vi "CheckValid.vi"(8 "error in (no error)":errorcluster, 11 "Cluster":T2) -> (0 "error out":errorcluster, 3 "Cluster 2":T1)   [LabVIEW 2019, in "lv-providershell-example2.lvlib"]
uses:
  lv-providershell-example2.lvlib
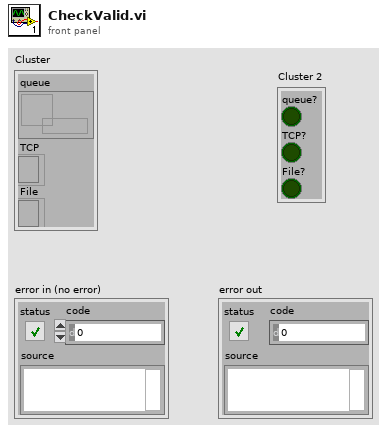
[diagram p1: front panel]
types:
  T1 = cluster{"queue?":bool, "TCP?":bool, "File?":bool}
  T2 = cluster{"queue":refnum<queue>, "TCP":refnum<k5>, "File":refnum<file>}
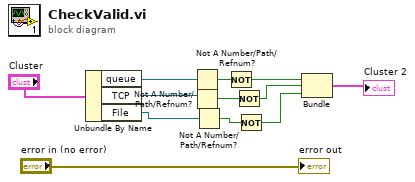
[diagram p0: block diagram]
diagram:
  n1 = Unbundle By Name("Cluster") -> ("queue"=w9:refnum<queue>, "TCP"=w8:refnum<k5>, "File"=w7:refnum<file>)
  n2 = Not A Number/Path/Refnum?(number/path/refnum=w9) -> (NaN/Path/Refnum?=w10:bool)
  n3 = Not A Number/Path/Refnum?(number/path/refnum=w8) -> (NaN/Path/Refnum?=w6:bool)
  n4 = Not A Number/Path/Refnum?(number/path/refnum=w7) -> (NaN/Path/Refnum?=w5:bool)
  n5 = Not(x=w10) -> (.not. x?=w4:bool)
  n6 = Not(x=w6) -> (.not. x?=w3:bool)
  n7 = Not(x=w5) -> (.not. x?=w2:bool)
  n8 = Bundle(w4, w3, w2) -> (→"Cluster 2":cluster{bool, bool, bool})  [unwired: 1 in]
  "error out" <- "error in (no error)"
